vi "testbed.vi"() -> ()   [LabVIEW 2023]
uses:
  <instrlib>/Agilent 34401/Public/Data/Read (Single Point).vi
  <instrlib>/Agilent 34401/Agilent 34401.lvlib
panel:
  out "Waveform Graph":dbl[](graph)
  out "Waveform Chart":dbl(graph)
  out "meaningless blinking light":bool
  out "Meter":dbl(knob) scale=0.0..10.0
  out "Measurement":dbl
  in  "Enable Auto Range (T: Enable)":bool=TRUE
  in  "Function (0: DC Voltage)":u16(ring) items=["DC Voltage", "AC Voltage", "2 - Wire Resistance", "4 - Wire Resistance", "DC Current", "AC Current", "Frequency", "Period", "Continuity", "Diode Checking", "VDC:VDC Ratio", "Temperature", "Capacitance"]
  out "Instrument Firmware Revision":string
  out "Instrument Driver Revision":string
  in  "VISA resource name":refnum<visa-resource-name>
  in  "milliseconds to wait":u32
  out "loop count":i32 format="%.2g"
  in  "want seconds? (F)":bool
  out "time string":string
  out "date string":string
  in  "Slide":dbl(slide) scale=0.0..10.0
  out "Thermometer":dbl(slide) scale=0.0..10.0
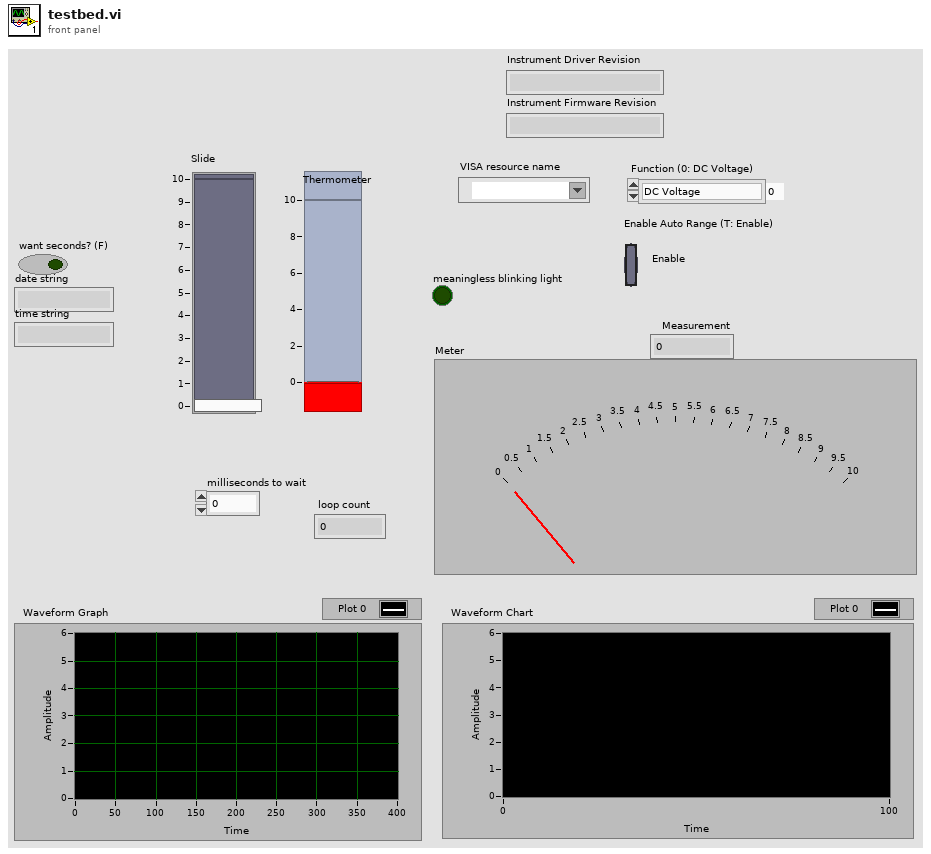
[diagram p1: front panel]
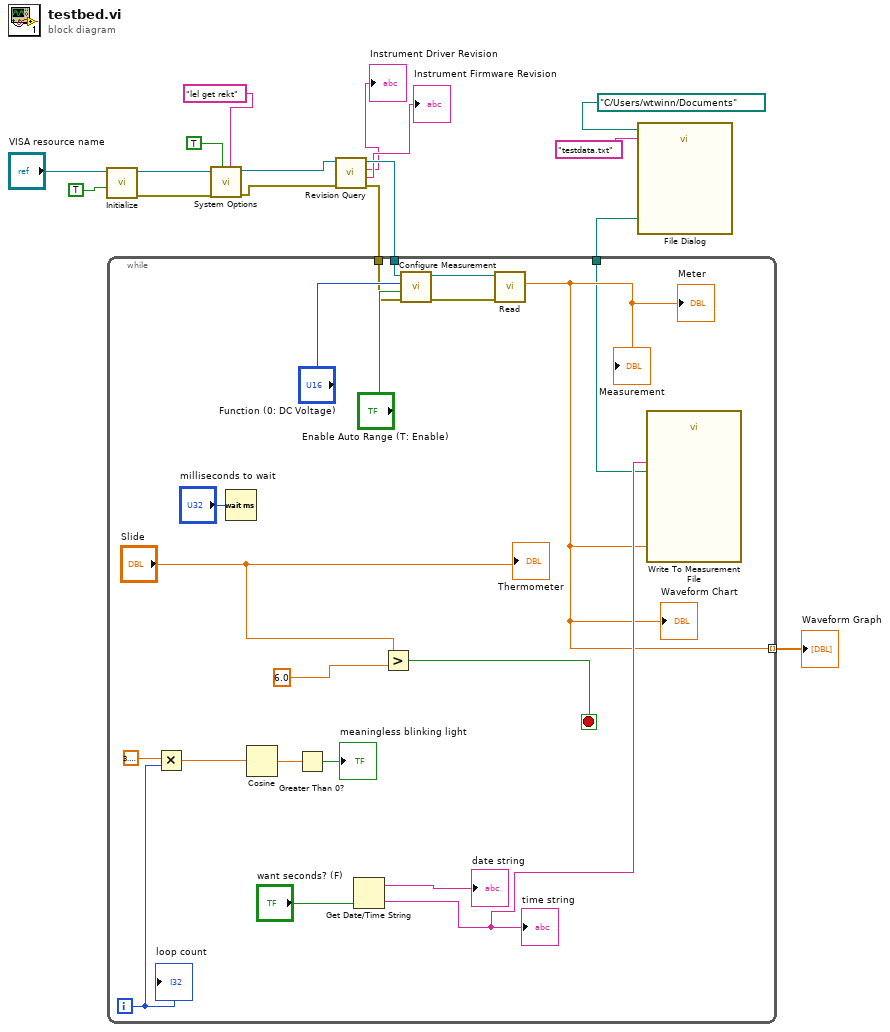
[diagram p0: block diagram]
diagram:
  n1 = call <instrlib>:"Initialize.vi"("Reset (True)"=TRUE, "VISA resource name"="VISA resource name") -> ("error out"=w14:errorcluster, "VISA resource name out"=w13:refnum<visa-resource-name>)  [unwired: 8 in]
  n2 = call <instrlib>:"System Options.vi"("Message Text (Empty)"="lel get rekt", "Message (F: Off)"=TRUE, "error in (no error)"=w14, "VISA resource name"=w13) -> ("error out"=w12:errorcluster, "VISA resource name out"=w11:refnum<visa-resource-name>)  [unwired: 6 in]
  n3 = call <instrlib>:"Revision Query.vi"("error in (no error)"=w12, "VISA resource name"=w11) -> ("error out"=w10:errorcluster, "Instrument Firmware Revision"=→"Instrument Firmware Revision":string, "Instrument Driver Revision"=→"Instrument Driver Revision":string, "VISA resource name out"=w9:refnum<visa-resource-name>)  [unwired: 6 in]
  n4 = call "File Dialog"("start path"=path "C:/Users/wtwinn/Documents", "default name"="testdata.txt") -> ("selected path"=w2:path)  [unwired: 10 in, 3 out]
  n5 = while {
    tunnel: w10 -> [w22]
    tunnel: w9 -> [w21]
    tunnel: w2 -> [w17]
    tunnel: [w18] -> w1 mode=indexing
    i -> [w28]
    stop <- w34 stop-if-true
    n6 = Multiply(x=3.141592653589793, y=w28) -> (x*y=w30:dbl)
    n7 = Wait (ms)(milliseconds to wait="milliseconds to wait") -> ()  [unwired: 1 out]
    n8 = Cosine(x=w30) -> (cos(x)=w27:dbl)
    n9 = Greater Than 0?(x=w27) -> (x > 0?=→"meaningless blinking light":bool)
    n10 = Get Date/Time String(want seconds? (F)="want seconds? (F)") -> (date string=→"date string":string, time string=w19:string)  [unwired: 2 in]
    "time string" <- w19
    n11 = Greater?(x="Slide", y=6.0) -> (0:w34:bool)
    n12 = call <instrlib>:"Configure Measurement.vi"("error in (no error)"=w22, "Enable Auto Range (T: Enable)"="Enable Auto Range (T: Enable)", "Function (0: DC Voltage)"="Function (0: DC Voltage)", "VISA resource name"=w21) -> ("error out"=w23:errorcluster, "VISA resource name out"=w24:refnum<visa-resource-name>)  [unwired: 6 in]
    n13 = call-poly <instrlib>:"Read.vi"("error in (no error)"=w23, "VISA resource name"=w24) -> ("Measurement"=w18:dbl)  [unwired: 7 in, 2 out]
    "Measurement" <- w18
    "Meter" <- w18
    "Waveform Chart" <- w18
    n14 = call "Write To Measurement File"("Signals"=w18, "Filename"=w17, "Comment"=w19) -> ()  [unwired: 14 in, 3 out]
    "Thermometer" <- "Slide"
    "loop count" <- w28
  }
  "Waveform Graph" <- w1
